vi "Level2a-Events.vi"() -> ()   [LabVIEW 2014]
doc: "Use this template to build a standard state machine design pattern. Each state executes code and determines which state to transition to. Contrast this design pattern with the User Interface Event Handler pattern, in which code executes in response to user actions. Contrast this design pattern also with the Queued Message Handler pattern, in which each message handling code can queue zero or more new messages."
uses:
  subVIs/Level2aState.ctl
panel:
  out "Current Time":timestamp format="%<%I:%M:%S %p\n%x>T"
  out "Input Data":dbl(graph)
  in  "Timer 2 Enabled":bool
  in  "Timer 1 Enabled":bool
  in  "Stop":bool
  out "Value > 0?":bool
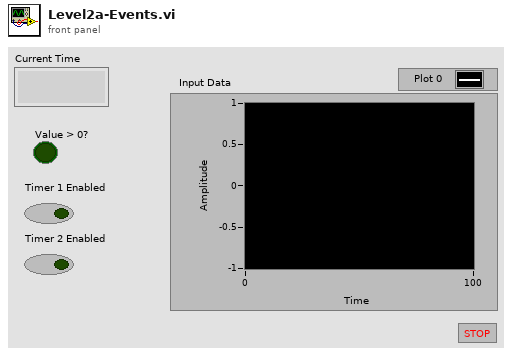
[diagram p1: front panel]
types:
  T1 = typedef "Level2aState.ctl" = enum16{"Check Inputs", "Check Clocks", "Clocks OnOff", "Generate Data", "Update Clock", "Stop"}
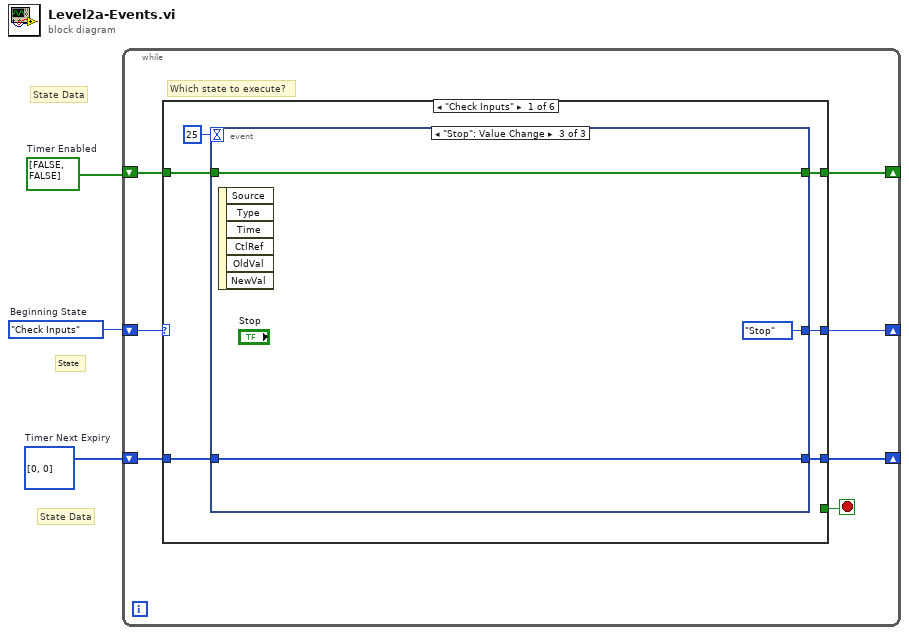
[diagram p0: block diagram]
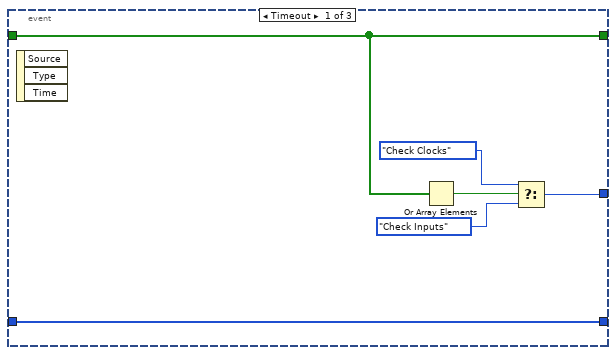
[diagram p2: hidden frame]
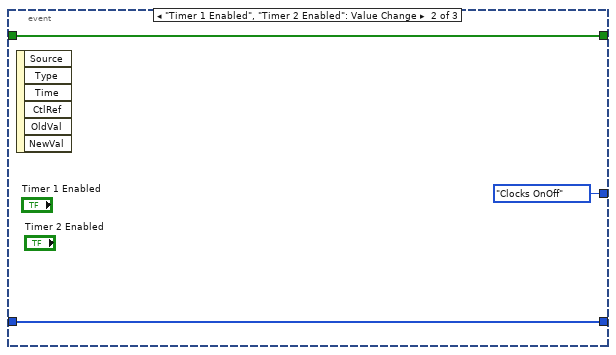
[diagram p3: hidden frame]
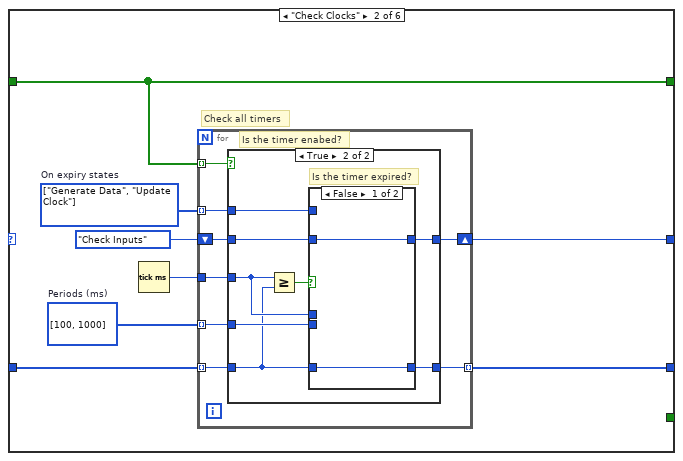
[diagram p4: hidden frame]
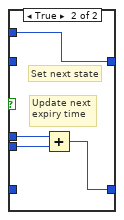
[diagram p6: hidden frame]
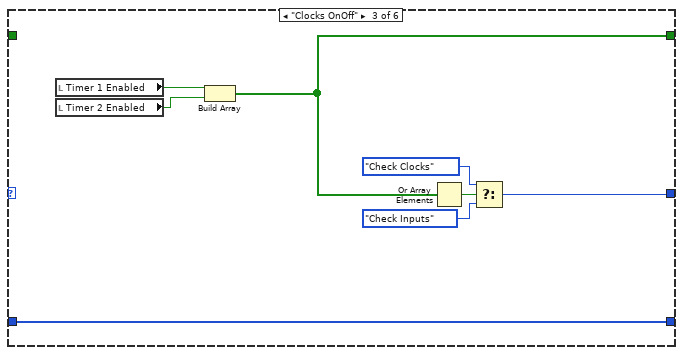
[diagram p7: hidden frame]
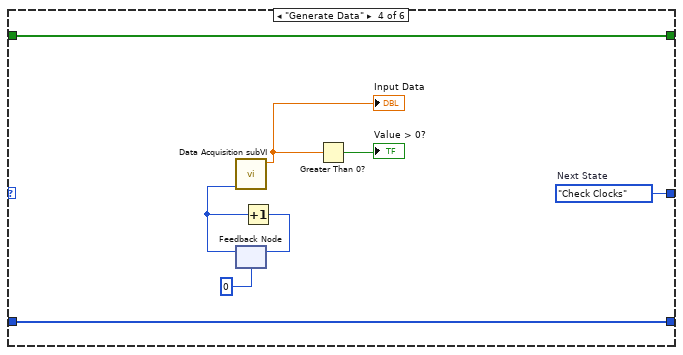
[diagram p8: hidden frame]
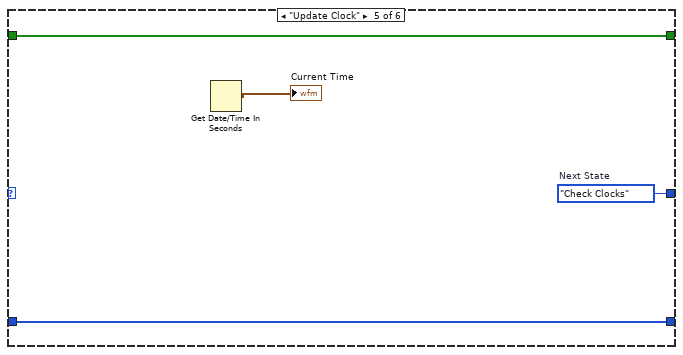
[diagram p9: hidden frame]
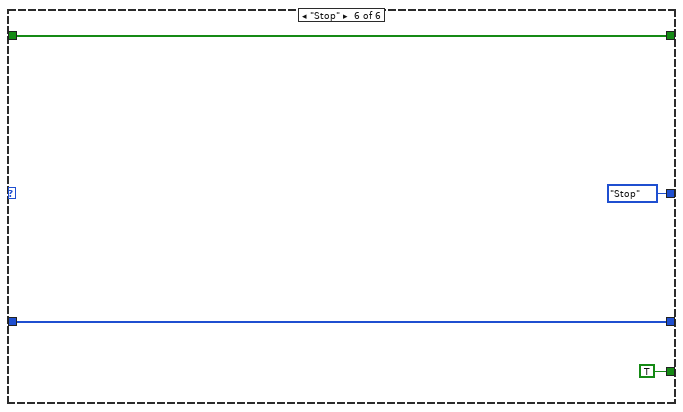
[diagram p10: hidden frame]
diagram:
  w1 = bool[] [FALSE, FALSE]  # Timer Enabled
  w2 = u32[] [0, 0]  # Timer Next Expiry
  w3 = Level2aState."Check Inputs"  # Beginning State
  # "State"
  # "State Data"
  # "State Data"
  n1 = while {
    shift-right: [w6] -> _
    shift-left: w3 -> [w9]
    shift-right: [w5] -> _
    shift-left: w2 -> [w10]
    shift-right: [w7] -> _
    shift-left: w1 -> [w8]
    stop <- w4 stop-if-true
    # "Which state to execute?"
    n2 = case shown="\"Check Inputs\"" w9 {
      tunnel: w10 -> [w11 w36 w61 w74 w79 w82]
      tunnel: w8 -> [w15 w35 _ w76 w80 w81]
      tunnel: [w13 w35 w66 w76 w80 w81] -> w7
      tunnel: [w16 w31 w62 w75 w78 Level2aState."Stop" ("Next State")] -> w6
      tunnel: [w12 w30 w61 w74 w79 w82] -> w5
      tunnel: [_ _ _ _ _ TRUE] -> w4
      frame "Check Inputs" {
        n3 = event shown="[2] \"Stop\": Value Change" {
          selector: _ -> [_ _ _]
          dyn-events: _ -> [_ _ _]
          timeout: 25 -> [_ _ _]
          tunnel: [w22 Level2aState."Clocks OnOff" ("States") Level2aState."Stop" ("States")] -> w16
          tunnel: w15 -> [w21 w25 w28]
          tunnel: [w21 w25 w28] -> w13
          tunnel: [w20 w24 w27] -> w12
          tunnel: w11 -> [w20 w24 w27]
          event Timeout {
            n4 = event-data() -> ()  [unwired: 1 in, 3 out]
            n5 = Or Array Elements(Boolean array=w21) -> (logical OR=w19:bool)
            n6 = Select(t=Level2aState."Check Clocks" ("States"), s=w19, f=Level2aState."Check Inputs" ("States")) -> (s? t:f=w22:T1)
          }
          event "Timer 1 Enabled", "Timer 2 Enabled": Value Change {
            n7 = event-data() -> ()  [unwired: 1 in, 6 out]
          }
          event "Stop": Value Change {
            n8 = event-data() -> ()  [unwired: 1 in, 6 out]
          }
        }
      }
      frame "Check Clocks" {
        w32 = T1[] [enum."Generate Data", enum."Update Clock"] items=["Check Inputs", "Check Clocks", "Clocks OnOff", "Generate Data", "Update Clock", "Stop"]  # On expiry states
        w33 = u32[] [100, 1000]  # Periods (ms)
        # "Check all timers"
        n9 = Tick Count (ms)() -> (millisecond timer value=w34:u32)
        n10 = for {
          tunnel: w36 -> [w42] mode=indexing
          tunnel: w35 -> [w44] mode=indexing
          tunnel: [w43] -> w30 mode=indexing
          shift-right: [w37] -> w31
          shift-left: Level2aState."Check Inputs" -> [w41]
          tunnel: w34 -> [w40]
          tunnel: w33 -> [w39] mode=indexing
          tunnel: w32 -> [w38] mode=indexing
          # "Is the timer enabed?"
          n11 = case shown="True" w44 {
            tunnel: [w46 w51] -> w43
            tunnel: w42 -> [w46 w50]
            tunnel: w41 -> [w45 w47]
            tunnel: w40 -> [_ w53]
            tunnel: w39 -> [_ w52]
            tunnel: w38 -> [_ w48]
            tunnel: [w45 w49] -> w37
            frame False {
              # "Timer disabled"
            }
            frame True {
              # "Is the timer expired?"
              n12 = Greater Or Equal?(x=w53, y=w50) -> (x >= y?=w54:bool)
              n13 = case shown="False" w54 {
                tunnel: w53 -> [_ w60]
                tunnel: w52 -> [_ w59]
                tunnel: [w56 w58] -> w51
                tunnel: w50 -> [w56 _]
                tunnel: [w55 w57] -> w49
                tunnel: w48 -> [_ w57]
                tunnel: w47 -> [w55 _]
                frame False {
                }
                frame True {
                  # "Set next state"
                  # "Update next\nexpiry time"
                  n14 = Add(x=w60, y=w59) -> (x+y=w58:u32)
                }
              }
            }
          }
        }
      }
      frame "Clocks OnOff" {
        n15 = local read "Timer 1 Enabled"() -> (w68:bool)
        n16 = local read "Timer 2 Enabled"() -> (w67:bool)
        n17 = Build Array(w68, w67) -> (w66:bool[])
        n18 = Or Array Elements(Boolean array=w66) -> (logical OR=w65:bool)
        n19 = Select(t=Level2aState."Check Clocks" ("Beginning State"), s=w65, f=Level2aState."Check Inputs" ("Beginning State")) -> (s? t:f=w62:T1)
      }
      frame "Generate Data" {
        w75 = Level2aState."Check Clocks"  # Next State
        n20 = feedback #1(0) -> (w71:i32)
        n21 = call "Data Acquisition subVI.vi"("Numeric in"=w71) -> ("Numeric out"=w70:dbl)  [unwired: 10 in]
        "Input Data" <- w70
        n22 = Increment(x=w71) -> (x+1=w73:i32)
        n23 = feedback-in #1(w73) -> ()
        n24 = Greater Than 0?(x=w70) -> (x > 0?=→"Value > 0?":bool)
      }
      frame "Update Clock" {
        w78 = Level2aState."Check Clocks"  # Next State
        n25 = Get Date/Time In Seconds() -> (seconds since 1Jan1904=→"Current Time":timestamp)
      }
      frame "Stop" {
      }
    }
  }
